vi "Read_Wrap_Simple.vi"(4 "Numeric in":refnum<class "Var_U16.lvclass">) -> (1 "Value":T1)   [LabVIEW 2021, in "Var_U16.lvclass"]
uses:
  Var_U16.lvclass
  Type.ctl
  Var_U16.lvclass/Var_U16.ctl
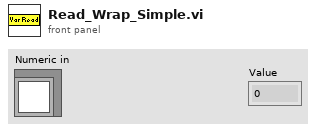
[diagram p1: front panel]
types:
  T1 = typedef "Var_U16.lvclass/Type.ctl" = dbl
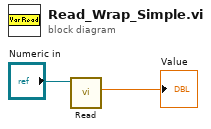
[diagram p0: block diagram]
diagram:
  n1 = call-dynamic "Read.vi"("Numeric in"="Numeric in") -> ("Numeric"=→"Value":T1)  [unwired: 8 in, 2 out]
